vi "Read Done.vi"(8 "error in (no error)":errorcluster, 9 "Bytes":u64, 10 "Time":dbl, 11 "Main in":refnum<class "Main.lvclass">) -> (0 "error out":errorcluster, 3 "Main out":refnum<class "Main.lvclass">)   [LabVIEW 2025, in "Main.lvlib" / "Main.lvclass"]
uses:
  Main.lvclass
  Main.lvclass/Main.ctl
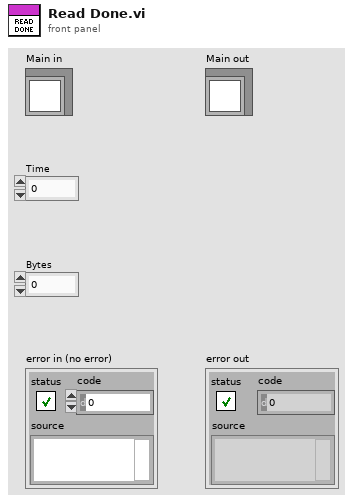
[diagram p1: front panel]
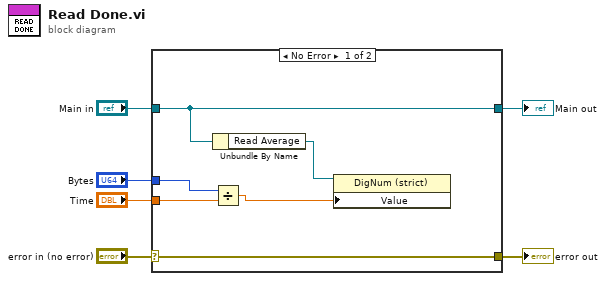
[diagram p0: block diagram]
diagram:
  n1 = case shown="No Error" "error in (no error)" {
    selector: "error in (no error)" -> [w12 w14]
    tunnel: [w12 w14] -> w5
    tunnel: [w9 w13] -> w3
    tunnel: "Main in" -> [w9 w13]
    tunnel: "Time" -> [w8 _]
    tunnel: "Bytes" -> [w7 _]
    frame No Error {
      n2 = Unbundle By Name(w9) -> ("Read Average"=w10:refnum<vi>)
      n3 = Divide(x=w7, y=w8) -> (x/y=w11:dbl)
      n4 = property class="DigNum (strict)"(reference=w10, "Value"=w11) -> ()  [unwired: 1 in, 2 out]
    }
    frame Error {
    }
  }
  "error out" <- w5
  "Main out" <- w3
